vi "ubinary_save_tagged.vi"(8 "error in":errorcluster, 9 "Tags":string[](array[string]), 10 "file (use dialog)":path, 11 "VI":refnum<vi>) -> (0 "error out":errorcluster)   [LabVIEW 2012]
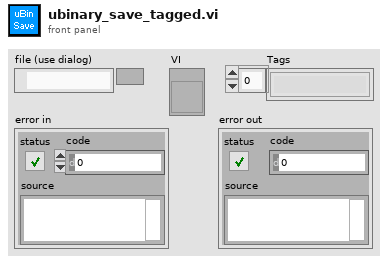
[diagram p1: front panel]
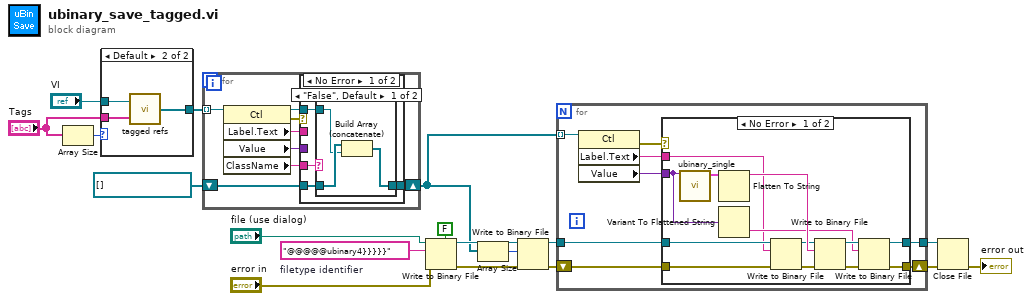
[diagram p0: block diagram]
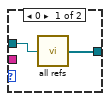
[diagram p2: hidden frame]
diagram:
  w12 = "@@@@@ubinary4}}}}}"  # filetype identifier
  n1 = Array Size(array="Tags") -> (size(s)=w2:i32)
  n2 = case shown="Default" w2 {
    tunnel: [w20 w21] -> w4
    tunnel: "VI" -> [w19 w23]
    tunnel: "Tags" -> [_ w22]
    frame 0 {
      n3 = call "all refs.vi"("VI"=w19) -> ("all controls"=w20:refnum<vi>[])
    }
    frame Default {
      n4 = call "tagged refs.vi"("Tags"=w22, "VI"=w23) -> ("tagged controls"=w21:refnum<vi>[])
    }
  }
  n5 = for {
    tunnel: w4 -> [w30] mode=indexing
    shift-right: [w26] -> w6
    shift-left: refnum<vi>[] [] ("ControlsOnPage") -> [w25]
    n6 = property class="Ctl"(reference=w30) -> (reference out=w24:refnum<vi>, error out=w31:errorcluster, "Label.Text"=w28:string, "Value"=w29:variant, "ClassName"=w27:string)  [unwired: 1 in]
    n7 = case shown="No Error" w31 {
      tunnel: w29 -> [_ _]
      tunnel: w28 -> [_ _]
      tunnel: w27 -> [w35 _]
      tunnel: [w33 w40] -> w26
      tunnel: w25 -> [w34 w40]
      tunnel: w24 -> [w32 _]
      frame No Error {
        n8 = case shown="\"False\", Default" w35 {
          tunnel: w34 -> [w38 w39]
          tunnel: [w36 w39] -> w33
          tunnel: w32 -> [w37 _]
          frame "False", Default {
            n9 = Build Array (concatenate)(w38, w37) -> (w36:refnum<vi>[])
          }
          frame "" {
          }
        }
      }
      frame Error {
      }
    }
  }
  n10 = Write to Binary File(file (use dialog)="file (use dialog)", data=w12, error in="error in", 5:FALSE ("prepend array or string size? (T)")) -> (refnum out=w13:refnum<file>, error out=w11:errorcluster)  [unwired: 2 in, 1 out]
  n11 = Array Size(array=w6) -> (size(s)=w5:i32)
  n12 = Write to Binary File(file (use dialog)=w13, data=w5, error in=w11) -> (refnum out=w15:refnum<file>, error out=w16:errorcluster)  [unwired: 3 in, 1 out]
  n13 = for {
    shift-right: [w47] -> w18
    shift-left: w16 -> [w44]
    tunnel: w15 -> [w45]
    tunnel: [w46] -> w17
    tunnel: w6 -> [w42] mode=indexing
    n14 = property class="Ctl"(reference=w42) -> (error out=w41:errorcluster, "Label.Text"=w43:string, "Value"=w48:variant)  [unwired: 1 in, 1 out]
    n15 = case shown="No Error" w41 {
      tunnel: w48 -> [w61 _]
      tunnel: [w57 w62] -> w47
      tunnel: [w55 w63] -> w46
      tunnel: w45 -> [w51 w63]
      tunnel: w44 -> [w50 w62]
      tunnel: w43 -> [w49 _]
      frame No Error {
        n16 = call "ubinary_single.vi"("Cluster"=w61) -> ("Header"=w60:cluster{"Element Names":string[], u8[]})  [unwired: 9 in, 1 out]
        n17 = Flatten To String(anything=w60) -> (data string=w59:string)  [unwired: 3 in, 2 out]
        n18 = Variant To Flattened String(Variant=w61) -> (data string=w54:string)  [unwired: 1 out]
        n19 = Write to Binary File(file (use dialog)=w51, data=w49, error in=w50) -> (refnum out=w52:refnum<file>, error out=w53:errorcluster)  [unwired: 3 in, 1 out]
        n20 = Write to Binary File(file (use dialog)=w52, data=w59, error in=w53) -> (refnum out=w56:refnum<file>, error out=w58:errorcluster)  [unwired: 3 in, 1 out]
        n21 = Write to Binary File(file (use dialog)=w56, data=w54, error in=w58) -> (refnum out=w55:refnum<file>, error out=w57:errorcluster)  [unwired: 3 in, 1 out]
      }
      frame Error {
      }
    }
  }
  n22 = Close File(refnum=w17, error in=w18) -> (error out=→"error out":errorcluster)  [unwired: 1 out]
